vi "uActor_Ping.vi"(8 "error in (no error)":errorcluster, 10 "timeout in ms (1000)":i32=1000, 11 "uActor Transport":refnum<class "uTransport_uActor.lvclass">) -> (0 "error out":errorcluster, 2 "latency (ms)":u32)   [LabVIEW 2023, in "uFramework.lvlib" / "uActor.lvclass"]
doc: "Pings the actor, to check if it is (1) initialized, (2) live, and (3) reactive to external messages.\nIt also measures the latency of the actor response, which may be used to check if a large buffer of queues messages is being consumed."
uses:
  uTransport_uActor/uTransport_uActor.lvclass
  uMsg/uMsg.lvclass/uMsg.ctl
  uTransport_uActor/uTransport_uActor.lvclass/uTransport_uActor.ctl
  uActor.lvclass
  uActor.lvclass/uActor.ctl
  uTransport/uTransport.lvclass
  <vilib>/ErrorRing/Error Ring.xnode
  U:/Projects/uFramework/Src/uFramework/uTransport_uActor/uTransport_uActor.lvclass
  U:/Projects/uFramework/Src/uFramework/uTransport/uTransport.lvclass
  <vilib>/Utility/error.llb/Error Cluster From Error Code.vi
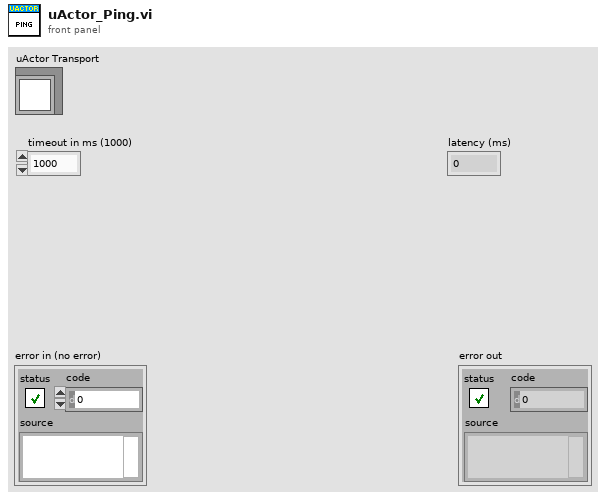
[diagram p1: front panel]
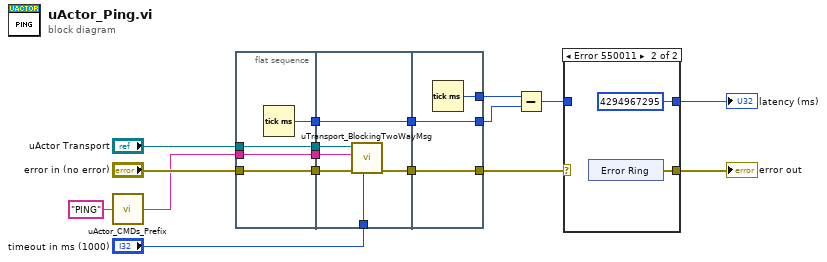
[diagram p0: block diagram]
diagram:
  n1 = call "uActor_CMDs_Prefix.vi"("uActor CMD"="PING") -> ("Reserved CMD"=w14:string)
  n2 = flat-sequence {
    tunnel: w14 -> [w19]
    tunnel: "error in (no error)" -> [w20]
    tunnel: "uActor Transport" -> [w21]
    tunnel: [w21] -> w12
    tunnel: [w20] -> w11
    tunnel: [w19] -> w10
    tunnel: [w18] -> w6
    tunnel: [w25] -> w13
    tunnel: w12 -> [w27]
    tunnel: w11 -> [w26]
    tunnel: w10 -> [w24]
    tunnel: [w23] -> w7
    tunnel: w6 -> [w23]
    tunnel: "timeout in ms (1000)" -> [w22]
    tunnel: [w30] -> w4
    tunnel: w13 -> [w30]
    tunnel: [w29] -> w9
    tunnel: [w28] -> w8
    tunnel: w7 -> [w28]
    frame #0 {
      n3 = Tick Count (ms)() -> (millisecond timer value=w18:u32)
    }
    frame #1 {
      n4 = call "uTransport_BlockingTwoWayMsg.vi"("timeout in ms (5000)"=w22, "error in (no error)"=w26, "Command"=w24, "uTransport in"=w27) -> ("error out"=w25:errorcluster)  [unwired: 6 in, 1 out]
    }
    frame #2 {
      n5 = Tick Count (ms)() -> (millisecond timer value=w29:u32)
    }
  }
  n6 = Subtract(x=w9, y=w8) -> (x-y=w1:u32)
  n7 = case shown="Error 550011" w4 {
    selector: w4 -> [w32 _]
    tunnel: [w32 w33] -> w3
    tunnel: [w31 u32 4294967295] -> w2
    tunnel: w1 -> [w31 _]
    frame #0 {
    }
    frame #1 {
      n8 = xnode "Error Ring"() -> ("error out"=w33:errorcluster)
    }
  }
  "error out" <- w3
  "latency (ms)" <- w2
